vi "Gear Delviery SS Controls to Commands 2017.vi"(11 "Pilot-CoPilot Controls":T2) -> (3 "Gear Delivery Commands":T1)   [LabVIEW 2016]
uses:
  Robot Control Outputs 2017.ctl
  Gear Delivery Commands.ctl
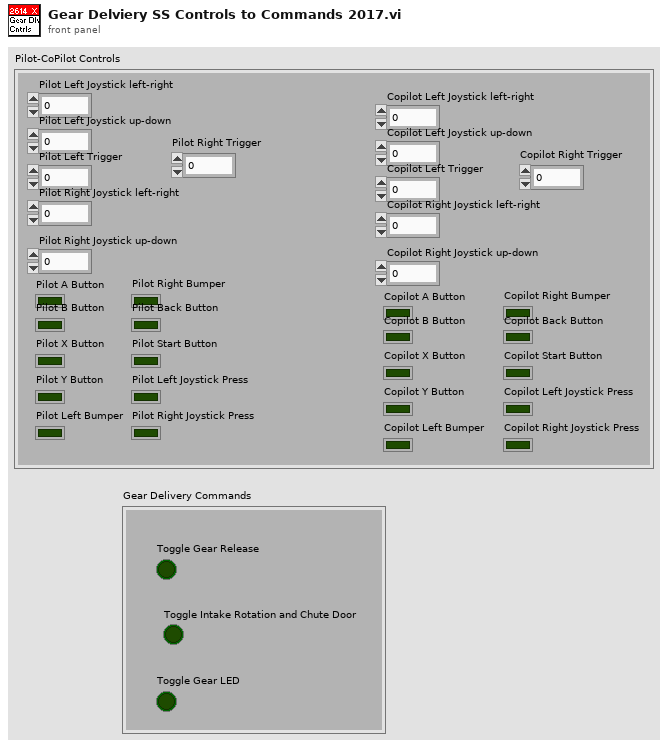
[diagram p1: front panel]
types:
  T1 = typedef "Gear Delivery Commands.ctl" = cluster{"Toggle Gear Release":bool, "Toggle Intake Rotation and Chute Door":bool, "Toggle Gear LED":bool}
  T2 = typedef "Robot Control Outputs 2017.ctl" = cluster{"Pilot Left Joystick left-right":dbl, "Pilot Left Joystick up-down":dbl, "Pilot A Button":bool, "Pilot B Button":bool, "Pilot X Button":bool, "Pilot Y Button":bool, "Pilot Left Bumper":bool, "Pilot Right Bumper":bool, "Pilot Back Button":bool, "Pilot Start Button":bool, "Pilot Left Joystick Press":bool, "Pilot Right Joystick Press":bool, "Pilot Left Trigger":dbl, "Pilot Right Joystick left-right":dbl, "Pilot Right Joystick up-down":dbl, "Pilot Right Trigger":dbl, "Copilot Left Joystick left-right":dbl, "Copilot Left Joystick up-down":dbl, "Copilot A Button":bool, "Copilot B Button":bool, "Copilot X Button":bool, "Copilot Y Button":bool, "Copilot Left Bumper":bool, "Copilot Right Bumper":bool, "Copilot Back Button":bool, "Copilot Start Button":bool, "Copilot Left Joystick Press":bool, "Copilot Right Joystick Press":bool, "Copilot Left Trigger":dbl, "Copilot Right Joystick left-right":dbl, "Copilot Right Joystick up-down":dbl, "Copilot Right Trigger":dbl}
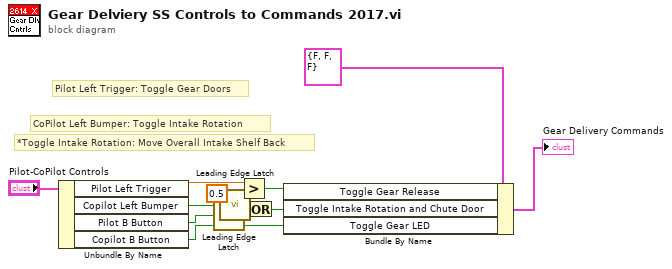
[diagram p0: block diagram]
diagram:
  # "*Toggle Intake Rotation: Move Overall Intake Shelf Back"
  # "CoPilot Left Bumper: Toggle Intake Rotation"
  # "Pilot Left Trigger: Toggle Gear Doors"
  n1 = Unbundle By Name("Pilot-CoPilot Controls") -> ("Pilot Left Trigger"=w9:dbl, "Copilot Left Bumper"=w6:bool, "Pilot B Button"=w2:bool, "Copilot B Button"=w5:bool)
  n2 = call "Leading Edge Latch.vi"("Input"=w2) -> ("Output"=w1:bool)
  n3 = call "Leading Edge Latch.vi"("Input"=w6) -> ("Output"=w4:bool)
  n4 = Greater?(x=w9, y=0.5) -> (0:w7:bool)
  n5 = Or(x=w4, y=w1) -> (x .or. y?=w3:bool)
  n6 = Bundle By Name(cluster=T1 {"Toggle Gear Release"=FALSE, "Toggle Intake Rotation and Chute Door"=FALSE, "Toggle Gear LED"=FALSE} ("Gear Delivery Commands"), "Toggle Gear Release"=w7, "Toggle Intake Rotation and Chute Door"=w3, "Toggle Gear LED"=w5) -> (→"Gear Delivery Commands":T1)
